vi "Controls State.vi"   [LabVIEW 2020, in "Enum Queue State Machine.lvlib"]
uses:
  Enum Queue State Machine.lvlib
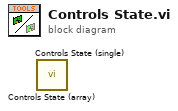
[diagram p0: block diagram]
diagram:
  n1 = call "Controls State (array).vi"() -> ()  [unwired: 11 in, 1 out]
  n2 = call "Controls State (single).vi"() -> ()  [unwired: 11 in, 1 out]
